vi "GetTerms4.vi"(0 "XRef":T12, 1 "State In":T10) -> (14 "Terms":T2, 15 "Fatal Error Out":T1)   [LabVIEW 2015, in "LVJSON.lvlib" / "Set Object Parameters.xnode"]
uses:
  Set Object Parameters.xnode
  <vilib>/XNodeSupport/XNodeXNodeRef.ctl
  State.ctl
  Get Object Parameters/Parameter.ctl
  <vilib>/XNodeSupport/XNodeTerm4Array.ctl
  <vilib>/XNodeSupport/XNodeTerm4.ctl
  <vilib>/XNodeSupport/XNodeString.ctl
  <vilib>/XNodeSupport/XNodeVariant.ctl
  <vilib>/XNodeSupport/XNodeRect32.ctl
  <vilib>/XNodeSupport/XNodeInt.ctl
  <vilib>/XNodeSupport/XNodeBool.ctl
  <vilib>/XNodeSupport/XNodeTermDirection.ctl
  <vilib>/XNodeSupport/XNodeErrorCluster.ctl
  JSON Object.lvclass
  JSON Numeric/JSON Numeric.lvclass
  JSON String/JSON String.lvclass
  JSON Boolean/JSON Boolean.lvclass
  JSON Datatype/JSON Null.lvclass
  JSON Array/JSON Array.lvclass
  offsets.vi
  <vilib>/XNodeSupport/NI_XNodeSupport.lvlib
  Shared/Shared.lvlib
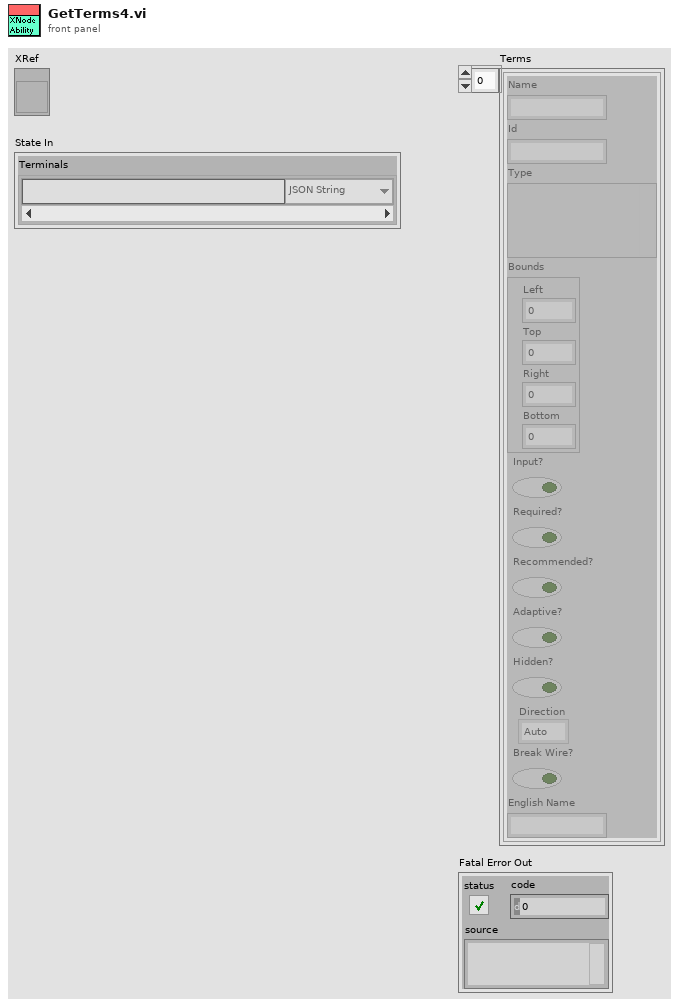
[diagram p1: front panel]
types:
  T1 = typedef "NI_XNodeSupport.lvlib/XNodeErrorCluster.ctl" = errorcluster
  T2 = typedef "NI_XNodeSupport.lvlib/XNodeTerm4Array.ctl" = T3[]
  T3 = typedef "NI_XNodeSupport.lvlib/XNodeTerm4.ctl" = cluster{"Name":T4, "Id":T4, "Type":T5, "Bounds":T6, "Input?":T8, "Required?":T8, "Recommended?":T8, "Adaptive?":T8, "Hidden?":T8, "Direction":T9, "Break Wire?":T8, "English Name":T4}
  T4 = typedef "NI_XNodeSupport.lvlib/XNodeString.ctl" = string
  T5 = typedef "NI_XNodeSupport.lvlib/XNodeVariant.ctl" = variant
  T6 = typedef "NI_XNodeSupport.lvlib/XNodeRect32.ctl" = cluster{"Left":T7, "Top":T7, "Right":T7, "Bottom":T7}
  T7 = typedef "NI_XNodeSupport.lvlib/XNodeInt.ctl" = i32
  T8 = typedef "NI_XNodeSupport.lvlib/XNodeBool.ctl" = bool
  T9 = typedef "NI_XNodeSupport.lvlib/XNodeTermDirection.ctl" = enum32{"Auto", "Up", "Down", "Left", "Right", "Center"}
  T10 = typedef "LVJSON.lvlib/Set Object Parameters.xnode/State.ctl" = cluster{"Terminals":T11[]}
  T11 = typedef "LVJSON.lvlib/Shared.lvlib/Parameter.ctl" = cluster{"Parameter Name":string, "JSON Type":enum16{"JSON String", "JSON Numeric", "JSON Boolean", "JSON", "JSON Object", "JSON Array", "String Value", "Numeric Value", "Boolean Value"}}
  T12 = typedef "NI_XNodeSupport.lvlib/XNodeXNodeRef.ctl" = refnum<vi>
  T13 = enum16{"JSON String", "JSON Numeric", "JSON Boolean", "JSON", "JSON Object", "JSON Array", "String Value", "Numeric Value", "Boolean Value"}
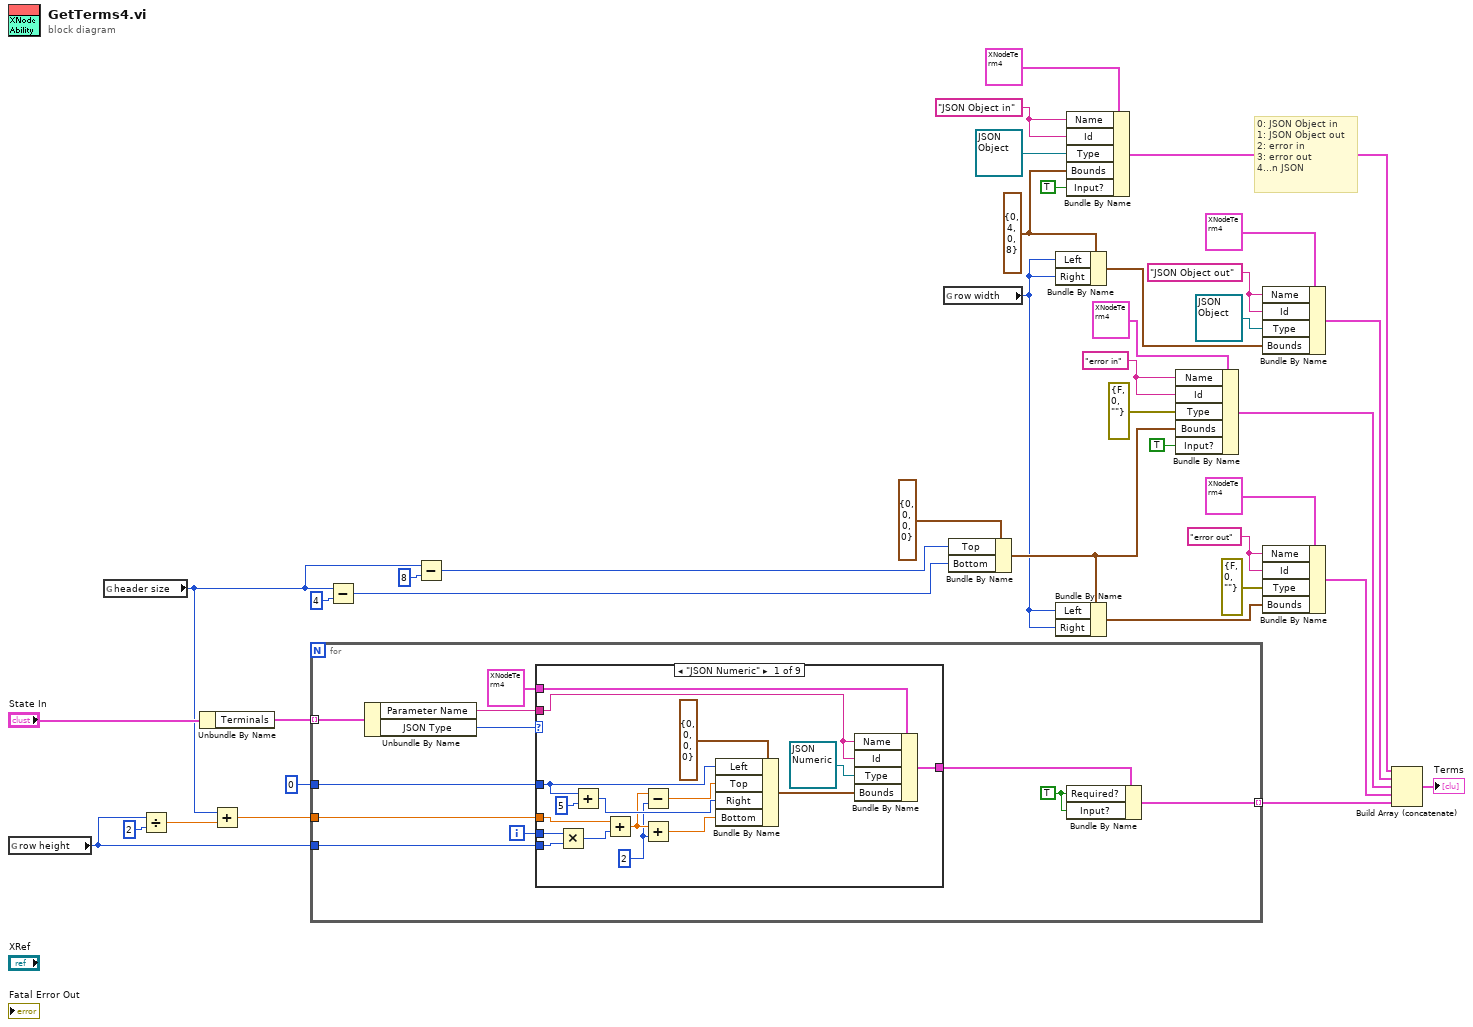
[diagram p0: block diagram]
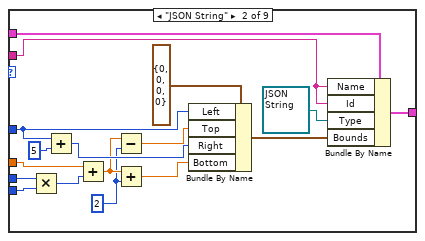
[diagram p2: hidden frame]
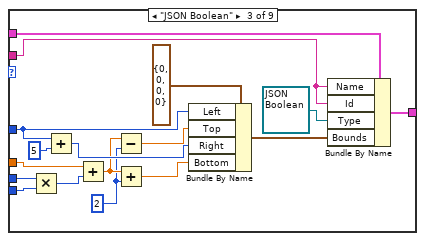
[diagram p3: hidden frame]
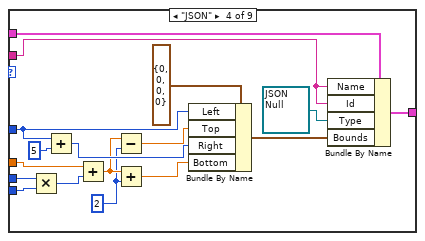
[diagram p4: hidden frame]
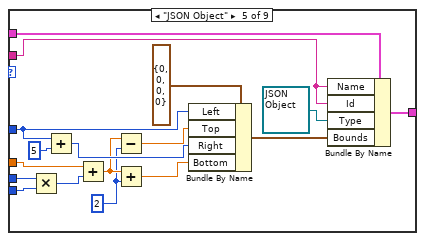
[diagram p5: hidden frame]
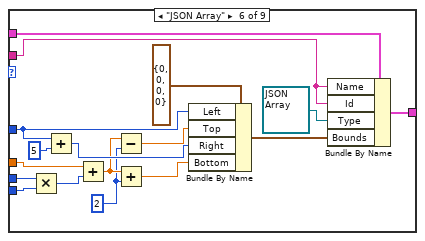
[diagram p6: hidden frame]
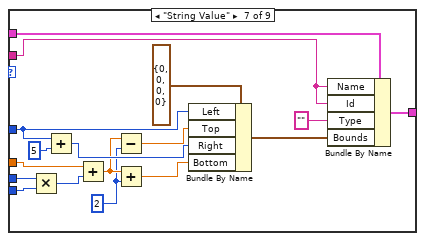
[diagram p7: hidden frame]
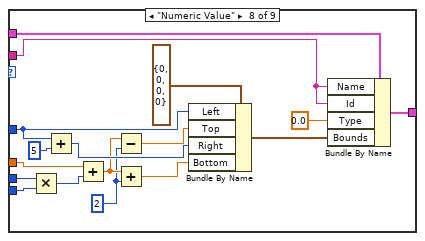
[diagram p8: hidden frame]
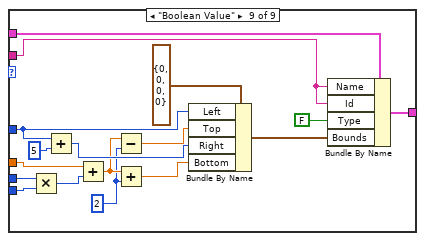
[diagram p9: hidden frame]
diagram:
  w10 = T4 "JSON Object out" ("Name")
  w7 = T6 {"Left"=0, "Top"=4, "Right"=0, "Bottom"=8} ("Bounds")
  w16 = T4 "JSON Object in" ("Name")
  w28 = T4 "error out" ("Name")
  w31 = T4 "error in" ("Name")
  # "0: JSON Object in\n1: JSON Object out\n2: error in\n3: error out\n4...n JSON"
  n1 = global read "offsets.vi" "row height"() -> (w36:i16)
  n2 = global read "offsets.vi" "header size"() -> (w25:i16)
  n3 = Divide(x=w36, y=i16 2) -> (x/y=w34:dbl)
  n4 = Unbundle By Name("State In") -> ("Terminals"=w37:T11[])
  n5 = Add(x=w25, y=w34) -> (x+y=w33:dbl)
  n6 = for {
    tunnel: w37 -> [w48] mode=indexing
    tunnel: w36 -> [w44]
    tunnel: w33 -> [w45]
    tunnel: i16 0 ("row width") -> [w42]
    tunnel: [w39] -> w1 mode=indexing
    i -> [w43]
    w40 = T8 TRUE ("Required?")
    n7 = Unbundle By Name(w48) -> ("Parameter Name"=w47:string, "JSON Type"=w46:T13)
    n8 = case shown="\"JSON Numeric\"" w46 {
      tunnel: T3 {"Name"="", "Id"="", "Type"=variant, "Bounds"={"Left"=0, "Top"=0, "Right"=0, "Bottom"=0}, "Input?"=FALSE, "Required?"=FALSE, "Recommended?"=FALSE, "Adaptive?"=FALSE, "Hidden?"=FALSE, "Direction"=enum."Auto", "Break Wire?"=FALSE, "English Name"=""} ("Term 4") -> [w66 w83 w100 w117 w134 w151 w168 w185 w202]
      tunnel: w47 -> [w53 w70 w87 w104 w121 w138 w156 w173 w190]
      tunnel: [w64 w81 w98 w115 w132 w149 w167 w184 w201] -> w41
      tunnel: w45 -> [w59 w76 w93 w110 w127 w144 w162 w179 w196]
      tunnel: w44 -> [w62 w79 w96 w113 w130 w147 w165 w182 w199]
      tunnel: w43 -> [w61 w78 w95 w112 w129 w146 w164 w181 w198]
      tunnel: w42 -> [w55 w72 w89 w106 w123 w140 w158 w175 w192]
      frame "JSON Numeric" {
        w51 = T7 2 ("Right")
        n9 = Multiply(x=w61, y=w62) -> (x*y=w60:i32)
        n10 = Add(x=w55, y=T7 5 ("Right")) -> (x+y=w54:T7)
        n11 = Add(x=w59, y=w60) -> (x+y=w52:dbl)
        n12 = Subtract(x=w52, y=w51) -> (x-y=w50:dbl)
        n13 = Add(x=w52, y=w51) -> (x+y=w58:dbl)
        n14 = Bundle By Name(cluster=T6 {"Left"=0, "Top"=0, "Right"=0, "Bottom"=0} ("Bounds"), "Left"=w55, "Top"=w50, "Right"=w54, "Bottom"=w58) -> (w57:T6)
        n15 = Bundle By Name(cluster=w66, "Name"=w53, "Id"=w53, "Type"=refnum<class "JSON Numeric.lvclass"> refnum ("JSON String out"), "Bounds"=w57) -> (w64:T3)
      }
      frame "JSON String" {
        w68 = T7 2 ("Right")
        n16 = Multiply(x=w78, y=w79) -> (x*y=w77:i32)
        n17 = Add(x=w72, y=T7 5 ("Right")) -> (x+y=w71:T7)
        n18 = Add(x=w76, y=w77) -> (x+y=w69:dbl)
        n19 = Subtract(x=w69, y=w68) -> (x-y=w67:dbl)
        n20 = Add(x=w69, y=w68) -> (x+y=w75:dbl)
        n21 = Bundle By Name(cluster=T6 {"Left"=0, "Top"=0, "Right"=0, "Bottom"=0} ("Bounds"), "Left"=w72, "Top"=w67, "Right"=w71, "Bottom"=w75) -> (w74:T6)
        n22 = Bundle By Name(cluster=w83, "Name"=w70, "Id"=w70, "Type"=refnum<class "JSON String.lvclass"> refnum ("JSON String out"), "Bounds"=w74) -> (w81:T3)
      }
      frame "JSON Boolean" {
        w85 = T7 2 ("Right")
        n23 = Multiply(x=w95, y=w96) -> (x*y=w94:i32)
        n24 = Add(x=w89, y=T7 5 ("Right")) -> (x+y=w88:T7)
        n25 = Add(x=w93, y=w94) -> (x+y=w86:dbl)
        n26 = Subtract(x=w86, y=w85) -> (x-y=w84:dbl)
        n27 = Add(x=w86, y=w85) -> (x+y=w92:dbl)
        n28 = Bundle By Name(cluster=T6 {"Left"=0, "Top"=0, "Right"=0, "Bottom"=0} ("Bounds"), "Left"=w89, "Top"=w84, "Right"=w88, "Bottom"=w92) -> (w91:T6)
        n29 = Bundle By Name(cluster=w100, "Name"=w87, "Id"=w87, "Type"=refnum<class "JSON Boolean.lvclass"> refnum ("JSON String out"), "Bounds"=w91) -> (w98:T3)
      }
      frame "JSON" {
        w102 = T7 2 ("Right")
        n30 = Multiply(x=w112, y=w113) -> (x*y=w111:i32)
        n31 = Add(x=w106, y=T7 5 ("Right")) -> (x+y=w105:T7)
        n32 = Add(x=w110, y=w111) -> (x+y=w103:dbl)
        n33 = Subtract(x=w103, y=w102) -> (x-y=w101:dbl)
        n34 = Add(x=w103, y=w102) -> (x+y=w109:dbl)
        n35 = Bundle By Name(cluster=T6 {"Left"=0, "Top"=0, "Right"=0, "Bottom"=0} ("Bounds"), "Left"=w106, "Top"=w101, "Right"=w105, "Bottom"=w109) -> (w108:T6)
        n36 = Bundle By Name(cluster=w117, "Name"=w104, "Id"=w104, "Type"=refnum<class "JSON Null.lvclass"> refnum ("JSON String out"), "Bounds"=w108) -> (w115:T3)
      }
      frame "JSON Object" {
        w119 = T7 2 ("Right")
        n37 = Multiply(x=w129, y=w130) -> (x*y=w128:i32)
        n38 = Add(x=w123, y=T7 5 ("Right")) -> (x+y=w122:T7)
        n39 = Add(x=w127, y=w128) -> (x+y=w120:dbl)
        n40 = Subtract(x=w120, y=w119) -> (x-y=w118:dbl)
        n41 = Add(x=w120, y=w119) -> (x+y=w126:dbl)
        n42 = Bundle By Name(cluster=T6 {"Left"=0, "Top"=0, "Right"=0, "Bottom"=0} ("Bounds"), "Left"=w123, "Top"=w118, "Right"=w122, "Bottom"=w126) -> (w125:T6)
        n43 = Bundle By Name(cluster=w134, "Name"=w121, "Id"=w121, "Type"=refnum<class "JSON Object.lvclass"> refnum ("JSON String out"), "Bounds"=w125) -> (w132:T3)
      }
      frame "JSON Array" {
        w136 = T7 2 ("Right")
        n44 = Multiply(x=w146, y=w147) -> (x*y=w145:i32)
        n45 = Add(x=w140, y=T7 5 ("Right")) -> (x+y=w139:T7)
        n46 = Add(x=w144, y=w145) -> (x+y=w137:dbl)
        n47 = Subtract(x=w137, y=w136) -> (x-y=w135:dbl)
        n48 = Add(x=w137, y=w136) -> (x+y=w143:dbl)
        n49 = Bundle By Name(cluster=T6 {"Left"=0, "Top"=0, "Right"=0, "Bottom"=0} ("Bounds"), "Left"=w140, "Top"=w135, "Right"=w139, "Bottom"=w143) -> (w142:T6)
        n50 = Bundle By Name(cluster=w151, "Name"=w138, "Id"=w138, "Type"=refnum<class "JSON Array.lvclass"> refnum ("JSON String out"), "Bounds"=w142) -> (w149:T3)
      }
      frame "String Value" {
        w154 = T7 2 ("Right")
        n51 = Multiply(x=w164, y=w165) -> (x*y=w163:i32)
        n52 = Add(x=w158, y=T7 5 ("Right")) -> (x+y=w157:T7)
        n53 = Add(x=w162, y=w163) -> (x+y=w155:dbl)
        n54 = Subtract(x=w155, y=w154) -> (x-y=w153:dbl)
        n55 = Add(x=w155, y=w154) -> (x+y=w161:dbl)
        n56 = Bundle By Name(cluster=T6 {"Left"=0, "Top"=0, "Right"=0, "Bottom"=0} ("Bounds"), "Left"=w158, "Top"=w153, "Right"=w157, "Bottom"=w161) -> (w160:T6)
        n57 = Bundle By Name(cluster=w168, "Name"=w156, "Id"=w156, "Type"="", "Bounds"=w160) -> (w167:T3)
      }
      frame "Numeric Value" {
        w171 = T7 2 ("Right")
        n58 = Multiply(x=w181, y=w182) -> (x*y=w180:i32)
        n59 = Add(x=w175, y=T7 5 ("Right")) -> (x+y=w174:T7)
        n60 = Add(x=w179, y=w180) -> (x+y=w172:dbl)
        n61 = Subtract(x=w172, y=w171) -> (x-y=w170:dbl)
        n62 = Add(x=w172, y=w171) -> (x+y=w178:dbl)
        n63 = Bundle By Name(cluster=T6 {"Left"=0, "Top"=0, "Right"=0, "Bottom"=0} ("Bounds"), "Left"=w175, "Top"=w170, "Right"=w174, "Bottom"=w178) -> (w177:T6)
        n64 = Bundle By Name(cluster=w185, "Name"=w173, "Id"=w173, "Type"=0.0, "Bounds"=w177) -> (w184:T3)
      }
      frame "Boolean Value" {
        w188 = T7 2 ("Right")
        n65 = Multiply(x=w198, y=w199) -> (x*y=w197:i32)
        n66 = Add(x=w192, y=T7 5 ("Right")) -> (x+y=w191:T7)
        n67 = Add(x=w196, y=w197) -> (x+y=w189:dbl)
        n68 = Subtract(x=w189, y=w188) -> (x-y=w187:dbl)
        n69 = Add(x=w189, y=w188) -> (x+y=w195:dbl)
        n70 = Bundle By Name(cluster=T6 {"Left"=0, "Top"=0, "Right"=0, "Bottom"=0} ("Bounds"), "Left"=w192, "Top"=w187, "Right"=w191, "Bottom"=w195) -> (w194:T6)
        n71 = Bundle By Name(cluster=w202, "Name"=w190, "Id"=w190, "Type"=FALSE, "Bounds"=w194) -> (w201:T3)
      }
    }
    n72 = Bundle By Name(cluster=w41, "Required?"=w40, "Input?"=w40) -> (w39:T3)
  }
  n73 = Subtract(x=w25, y=i16 4) -> (x-y=w22:i16)
  n74 = Subtract(x=w25, y=i16 8) -> (x-y=w21:i16)
  n75 = global read "offsets.vi" "row width"() -> (w2:i16)
  n76 = Bundle By Name(cluster=T6 {"Left"=0, "Top"=0, "Right"=0, "Bottom"=0} ("Bounds"), "Top"=w21, "Bottom"=w22) -> (w20:T6)
  n77 = Bundle By Name(cluster=w7, "Left"=w2, "Right"=w2) -> (w6:T6)
  n78 = Bundle By Name(cluster=w20, "Left"=w2, "Right"=w2) -> (w19:T6)
  n79 = Bundle By Name(cluster=T3 {"Name"="", "Id"="", "Type"=variant, "Bounds"={"Left"=0, "Top"=0, "Right"=0, "Bottom"=0}, "Input?"=FALSE, "Required?"=FALSE, "Recommended?"=FALSE, "Adaptive?"=FALSE, "Hidden?"=FALSE, "Direction"=enum."Auto", "Break Wire?"=FALSE, "English Name"=""} ("Term 4"), "Name"=w16, "Id"=w16, "Type"=refnum<class "JSON Object.lvclass"> refnum ("JSON String out"), "Bounds"=w7, "Input?"=T8 TRUE) -> (w5:T3)
  n80 = Bundle By Name(cluster=T3 {"Name"="", "Id"="", "Type"=variant, "Bounds"={"Left"=0, "Top"=0, "Right"=0, "Bottom"=0}, "Input?"=FALSE, "Required?"=FALSE, "Recommended?"=FALSE, "Adaptive?"=FALSE, "Hidden?"=FALSE, "Direction"=enum."Auto", "Break Wire?"=FALSE, "English Name"=""} ("Term 4"), "Name"=w31, "Id"=w31, "Type"=errorcluster {"status"=FALSE, "code"=0, "source"=""} ("error constant"), "Bounds"=w20, "Input?"=T8 TRUE) -> (w18:T3)
  n81 = Bundle By Name(cluster=T3 {"Name"="", "Id"="", "Type"=variant, "Bounds"={"Left"=0, "Top"=0, "Right"=0, "Bottom"=0}, "Input?"=FALSE, "Required?"=FALSE, "Recommended?"=FALSE, "Adaptive?"=FALSE, "Hidden?"=FALSE, "Direction"=enum."Auto", "Break Wire?"=FALSE, "English Name"=""} ("Term 4"), "Name"=w10, "Id"=w10, "Type"=refnum<class "JSON Object.lvclass"> refnum ("JSON String out"), "Bounds"=w6) -> (w4:T3)
  n82 = Bundle By Name(cluster=T3 {"Name"="", "Id"="", "Type"=variant, "Bounds"={"Left"=0, "Top"=0, "Right"=0, "Bottom"=0}, "Input?"=FALSE, "Required?"=FALSE, "Recommended?"=FALSE, "Adaptive?"=FALSE, "Hidden?"=FALSE, "Direction"=enum."Auto", "Break Wire?"=FALSE, "English Name"=""} ("Term 4"), "Name"=w28, "Id"=w28, "Type"=errorcluster {"status"=FALSE, "code"=0, "source"=""} ("error constant"), "Bounds"=w19) -> (w17:T3)
  n83 = Build Array (concatenate)(w5, w4, w18, w17, w1) -> (→"Terms":T3[])
